vi "StringToCDB[](cast).vi"(1 "String":string) -> (0 "CDB[]":cdb[](array[numeric]))   [LabVIEW 2012]
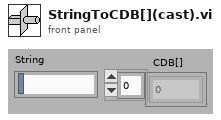
[diagram p1: front panel]
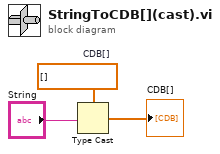
[diagram p0: block diagram]
diagram:
  w2 = cdb[] []  # CDB[]
  n1 = Type Cast(type=w2, x="String") -> (*(type *) &x=→"CDB[]":cdb[])
